vi "Enable Source Read Back.vi"(8 "error in (no error)":errorcluster, 9 "Enable Read Back  (T:Enable)":bool=TRUE, 10 "Function (0: Volts)":u16(ring) items=["Volts", "Current"], 11 "VISA resource name":refnum<visa-resource-name>) -> (0 "error out":errorcluster, 3 "VISA resource name out":refnum<visa-resource-name>)   [LabVIEW 2018, in "Keithley 2450.lvlib"]
doc: "Enable or disable source read back on the instrument for the selected function."
uses:
  <instrlib>/Keithley 2450/Keithley 2450.lvlib
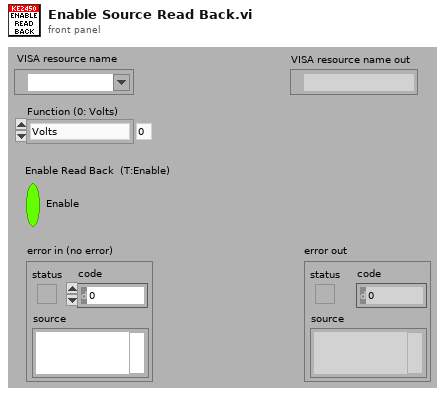
[diagram p1: front panel]
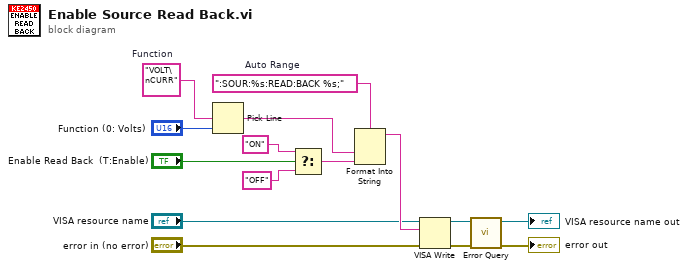
[diagram p0: block diagram]
diagram:
  w5 = "VOLT\nCURR"  # Function
  w11 = ":SOUR:%s:READ:BACK %s;"  # Auto Range
  n1 = Pick Line(multi-line string=w5, line index="Function (0: Volts)") -> (output string=w3:string)  [unwired: 1 out]
  n2 = Select(t="ON", s="Enable Read Back  (T:Enable)", f="OFF") -> (s? t:f=w8:string)
  n3 = Format Into String(format string=w11, w3, w8) -> (resulting string=w7:string)  [unwired: 2 in, 1 out]
  n4 = VISA Write(VISA resource name="VISA resource name", write buffer=w7, error in (no error)="error in (no error)") -> (VISA resource name out=w13:refnum<visa-resource-name>, error out=w12:errorcluster)  [unwired: 1 out]
  n5 = call <instrlib>:"Error Query.vi"("error in (no error)"=w12, "VISA resource name"=w13) -> ("error out"=→"error out":errorcluster, "VISA resource name out"=→"VISA resource name out":refnum<visa-resource-name>)  [unwired: 8 out]
